vi "Shooter Teleop Handler.vi"() -> ()   [LabVIEW 2025]
uses:
  <vilib>/Rock Robotics/WPI/Joystick/XBox Buttons Indexer.ctl
  <vilib>/Rock Robotics/WPI/Joystick/XBox Axes Indexer.ctl
  <vilib>/Rock Robotics/WPI/Utilities/WPI_GetSetVariantRefNum.vi
  <vilib>/Rock Robotics/WPI/ThirdParty/REV Robotics/REVLib/SubVI/Public/SPARK Get Encoder Status Velocity.vi
  Framework/Robot Global Data.vi
panel:
  out "Distance to hub":dbl=8.933713100095792
  in  "Outtake":dbl=-0.75
  in  "Interp\nLPK":dbl=5500.0
  in  "Interp TS":dbl=0.65
  in  "Interp UPK":dbl=5000.0
  in  "Idle Speeds":T1={"Hood Setpoint"=0.0, "UPK"=0.0, "Flywheel"=1000.0, "LPK"=0.0, "Transfer Speed"=0.0}
  in  "Preset Speeds":T1={"Hood Setpoint"=4200.0, "UPK"=5500.0, "Flywheel"=4000.0, "LPK"=5000.0, "Transfer Speed"=0.65}
  in  "Manual  Speeds":T1={"Hood Setpoint"=0.0, "UPK"=0.0, "Flywheel"=0.0, "LPK"=0.0, "Transfer Speed"=0.65}
  in  "Manual Overrides?":bool
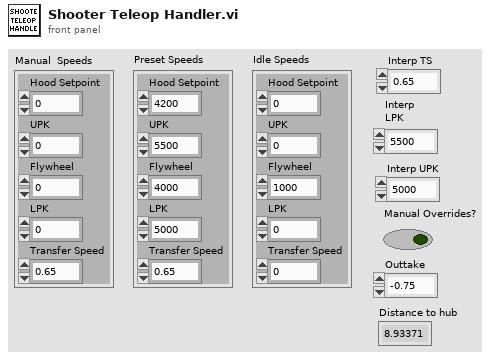
[diagram p1: front panel]
types:
  T1 = cluster{"Hood Setpoint":dbl, "UPK":dbl, "Flywheel":dbl, "LPK":dbl, "Transfer Speed":dbl}
  T2 = typedef "XBox Axes Indexer.ctl" = enum16{"Left X", "Left Y", "Left Trigger", "Right Trigger", "Right X", "Right Y"}
  T3 = typedef "XBox Buttons Indexer.ctl" = enum16{"A", "B", "X", "Y", "Left Bumper", "Right Bumper", "Back", "Start", "Left Joystick", "Right Joystick"}
  T4 = typedef "WPI_JoystickDevRef.ctl" = cluster{"Device":T5}
  T5 = typedef "WPI_JoystickDeviceEnum.ctl" = enum16{"USB 0", "USB 1", "USB 2", "USB 3", "USB 4", "USB 5"}
  T6 = typedef "WPI_MotorControlDeviceRef.ctl" = cluster{"DeviceStatus":errorcluster, "Type":T7, "PWM":cluster{"PWM Channel":T8, "DeadBand":T9}, "CAN":cluster{"Device Number":u8, "SetOutput VI Ref":variant, "GetOutput VI Ref":variant, "Enable VI Ref":variant, "Disable VI Ref":variant, "Data":variant}, "Invert":bool, "DIO PWM":cluster{"PWM \"Enable\" Channel":T8, "DIOChannel":T10, "PWM Rate":dbl}}
  T7 = typedef "WPI_MotorControlType.ctl" = enum16{"PWM", "CAN", "DIO PWM"}
  T8 = typedef "FPGA_DIOPWMChannel.ctl" = enum8{"PWM 0", "PWM 1", "PWM 2", "PWM 3", "PWM 4", "PWM 5", "PWM 6", "PWM 7", "PWM 8", "PWM 9", "PWM MXP 0", "PWM MXP 1", "PWM MXP 2", "PWM MXP 3", "PWM MXP 4", "PWM MXP 5", "PWM MXP 6", "PWM MXP 7", "PWM MXP 8", "PWM MXP 9", "Invalid"}
  T9 = typedef "WPI_PWMDeadband.ctl" = cluster{"Name":string, "maxPositivePwm":i32, "minPositivePwm":i32, "centerPwm":i32, "maxNegativePwm":i32, "minNegativePwm":i32, "angularRange":u16}
  T10 = typedef "FPGA_DIOChannel.ctl" = enum8{"DIO 0", "DIO 1", "DIO 2", "DIO 3", "DIO 4", "DIO 5", "DIO 6", "DIO 7", "DIO 8", "DIO 9", "DIO MXP 0", "DIO MXP 1", "DIO MXP 2", "DIO MXP 3", "DIO MXP 4", "DIO MXP 5", "DIO MXP 6", "DIO MXP 7", "DIO MXP 8", "DIO MXP 9", "DIO MXP 10", "DIO MXP 11", "DIO MXP 12", "DIO MXP 13", "DIO MXP 14", "DIO MXP 15", "SPI Port CS1", "SPI Port CS2", "SPI Port CS3", "SPI Port MISO", "SPI Port MOSI", "Invalid"}
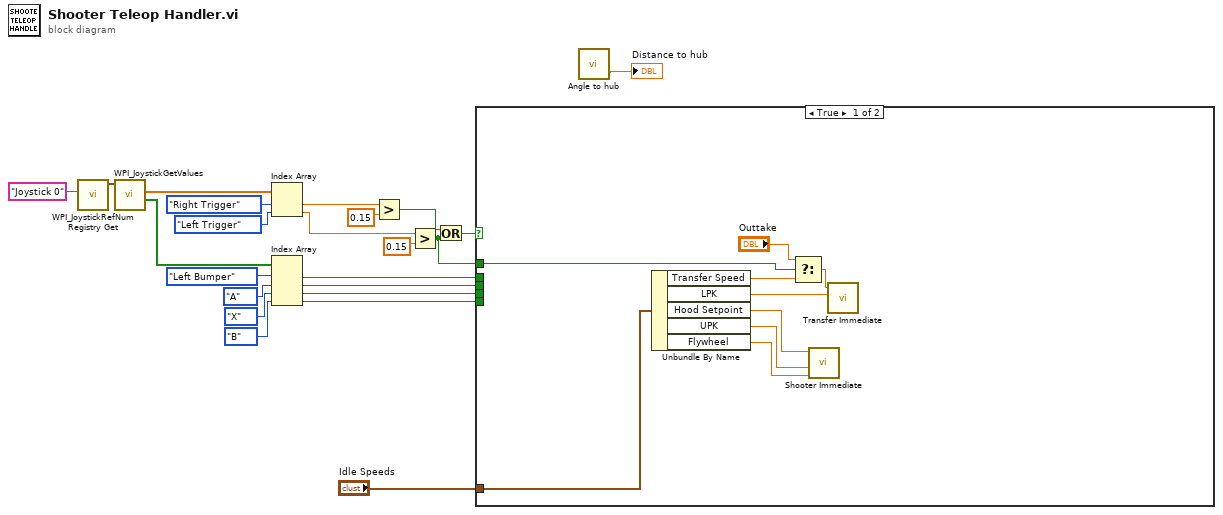
[diagram p0: block diagram]
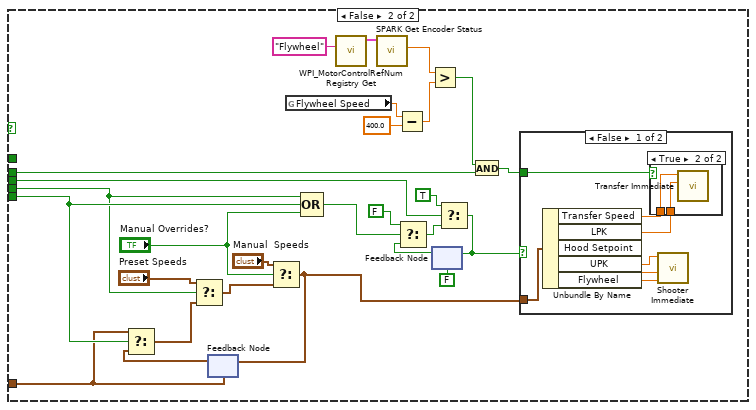
[diagram p2: hidden frame]
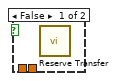
[diagram p3: hidden frame]
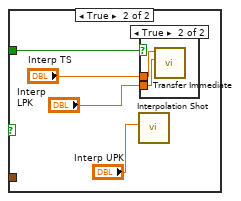
[diagram p4: hidden frame]
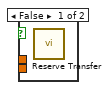
[diagram p5: hidden frame]
diagram:
  n1 = call <vilib>:"WPI_JoystickRefNum Registry Get.vi"("refnum name"="Joystick 0") -> ("JoystickDevRef"=w22:T4)  [unwired: 1 in, 9 out]
  n2 = call <vilib>:"WPI_JoystickGetValues.vi"("JoystickDevRef"=w22) -> ("Buttons"=w20:bool[], "Axes"=w21:dbl[])  [unwired: 6 in, 3 out]
  n3 = Index Array(array=w21, index #1=XBox_Axes_Indexer."Right Trigger" ("XBox Axes"), index #2=XBox_Axes_Indexer."Left Trigger" ("XBox Axes")) -> (element #1=w16:dbl, element #2=w4:dbl)
  n4 = Index Array(array=w20, index #1=XBox_Buttons_Indexer."Left Bumper" ("XBox Buttons"), index #2=XBox_Buttons_Indexer."A" ("XBox Buttons"), index #3=XBox_Buttons_Indexer."X" ("XBox Buttons"), index #4=XBox_Buttons_Indexer."B" ("XBox Buttons")) -> (element #1=w9:bool, element #2=w13:bool, element #3=w12:bool, element #4=w11:bool)
  n5 = Greater?(x=w16, y=0.15) -> (0:w7:bool)
  n6 = Greater?(x=w4, y=0.15) -> (0:w3:bool)
  n7 = Or(x=w7, y=w3) -> (x .or. y?=w8:bool)
  n8 = case shown="True" w8 {
    tunnel: w13 -> [_ w49]
    tunnel: w12 -> [_ w38]
    tunnel: w11 -> [_ w39]
    tunnel: w9 -> [_ w34]
    tunnel: w3 -> [w26 _]
    tunnel: "Idle Speeds" -> [w24 w33]
    frame True {
      n9 = Unbundle By Name(w24) -> ("Transfer Speed"=w27:dbl, "LPK"=w32:dbl, "Hood Setpoint"=w31:dbl, "UPK"=w30:dbl, "Flywheel"=w29:dbl)
      n10 = Select(t="Outtake", s=w26, f=w27) -> (s? t:f=w28:dbl)
      n11 = call "Shooter Immediate.vi"("Flywheel Setpoint"=w29, "Upper Kicker Setpoint"=w30, "Hood Setpoint"=w31) -> ()  [unwired: 6 in, 1 out]
      n12 = call "Transfer Immediate.vi"("Lower Kicker Speed"=w32, "Transfer Speed"=w28) -> ()  [unwired: 9 in, 1 out]
    }
    frame False {
      n13 = feedback #1(w33) -> (w55:T1)
      n14 = Select(t=w33, s=w39, f=w55) -> (s? t:f=w56:T1)
      n15 = Select(t="Preset Speeds", s=w38, f=w56) -> (s? t:f=w57:T1)
      n16 = Select(t="Manual  Speeds", s="Manual Overrides?", f=w57) -> (s? t:f=w47:T1)
      n17 = feedback-in #1(w47) -> ()
      n18 = global read "Robot Global Data.vi" "Flywheel Speed"() -> (w46:dbl)
      n19 = Compound Arithmetic op=OR(w38, w39, "Manual Overrides?") -> (w37:bool)
      n20 = call <vilib>:"WPI_MotorControlRefNum Registry Get.vi"("refnum name"="Flywheel") -> ("MotorControlDevRef"=w41:T6)  [unwired: 9 in, 1 out]
      n21 = call-poly <vilib>:"SPARK Get Encoder Status.vi"("MotorControlDevRef in"=w41) -> ("Sensor Velocity"=w44:dbl)  [unwired: 7 in, 3 out]
      n22 = Subtract(x=w46, y=400.0) -> (x-y=w45:dbl)
      n23 = Greater?(x=w44, y=w45) -> (0:w35:bool)
      n24 = feedback #2(FALSE ("t")) -> (w51:bool)
      n25 = Select(t=FALSE, s=w37, f=w51) -> (s? t:f=w53:bool)
      n26 = Select(t=TRUE, s=w49, f=w53) -> (s? t:f=w48:bool)
      n27 = feedback-in #2(w48) -> ()
      n28 = And(x=w35, y=w34) -> (x .and. y?=w36:bool)
      n29 = case shown="False" w48 {
        tunnel: w47 -> [w65 _]
        tunnel: w36 -> [w66 w71]
        frame False {
          n30 = Unbundle By Name(w65) -> ("Transfer Speed"=w64:dbl, "LPK"=w63:dbl, "Hood Setpoint"=w62:dbl, "UPK"=w61:dbl, "Flywheel"=w60:dbl)
          n31 = case shown="True" w66 {
            tunnel: w64 -> [_ w68]
            tunnel: w63 -> [_ w67]
            frame False {
              n32 = call "Reserve Transfer.vi"() -> ()  [unwired: 11 in, 1 out]
            }
            frame True {
              n33 = call "Transfer Immediate.vi"("Lower Kicker Speed"=w67, "Transfer Speed"=w68) -> ()  [unwired: 9 in, 1 out]
            }
          }
          n34 = call "Shooter Immediate.vi"("Flywheel Setpoint"=w60, "Upper Kicker Setpoint"=w61, "Hood Setpoint"=w62) -> ()  [unwired: 6 in, 1 out]
        }
        frame True {
          n35 = call "Interpolation Shot.vi"("Upper Kicker Setpoint"="Interp UPK") -> ()  [unwired: 10 in, 1 out]
          n36 = case shown="True" w71 {
            tunnel: "Interp TS" -> [_ w74]
            tunnel: "Interp\nLPK" -> [_ w73]
            frame False {
              n37 = call "Reserve Transfer.vi"() -> ()  [unwired: 11 in, 1 out]
            }
            frame True {
              n38 = call "Transfer Immediate.vi"("Lower Kicker Speed"=w73, "Transfer Speed"=w74) -> ()  [unwired: 9 in, 1 out]
            }
          }
        }
      }
    }
  }
  n39 = call "Angle to hub.vi"() -> ("Distance to hub"=→"Distance to hub":dbl)  [unwired: 2 in, 1 out]
